vi "Destroy.vi"(8 "error in (no error)":errorcluster, 9 "ms Timeout (500)":u32=500, 11 "Queue in":refnum<queue>) -> (0 "error out":errorcluster, 1 "ms Elapsed":u32, 3 "Queue out":refnum<queue>)   [LabVIEW 2021, in "QueueTimer.lvlib"]
doc: "Destroys all queue timers associated with the <b>Queue</b> reference and stops the daemon threads. Specify the <b>ms Timeout</b> to wait for the daemon thread to close.\n\nNote: The Wait on Async is used which hardcodes the timeout values, supported timeout values are 0ms (No wait), 500ms, 2000ms and 5000ms."
uses:
  QueueTimer.lvlib
  <vilib>/Utility/error.llb/Error Cluster From Error Code.vi
  <vilib>/ErrorRing/Error Ring.xnode
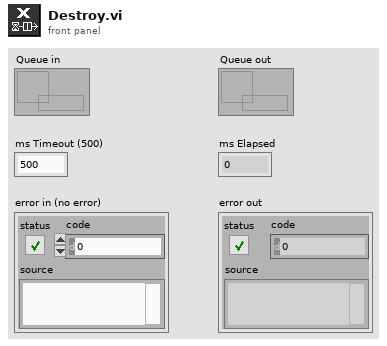
[diagram p1: front panel]
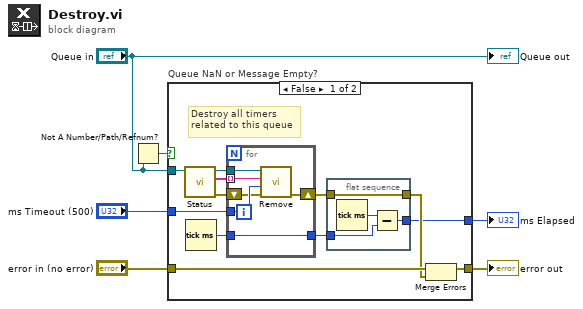
[diagram p0: block diagram]
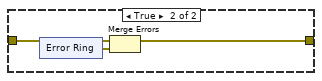
[diagram p2: hidden frame]
diagram:
  n1 = Not A Number/Path/Refnum?(number/path/refnum="Queue in") -> (NaN/Path/Refnum?=w3:bool)
  n2 = case "Queue NaN or Message Empty?" shown="False" w3 {
    tunnel: "Queue in" -> [w17 _]
    tunnel: "error in (no error)" -> [w10 w31]
    tunnel: [w13 w30] -> w5
    tunnel: "ms Timeout (500)" -> [w18 _]
    tunnel: [w7 _] -> w2
    frame False {
      # "Destroy all timers\nrelated to this queue"
      n3 = call "Status.vi"("Queue in"=w17) -> ("error out"=w15:errorcluster, "Timer Messages"=w14:string[], "Queue out"=w16:refnum<queue>)  [unwired: 5 in, 3 out]
      n4 = Tick Count (ms)() -> (millisecond timer value=w12:u32)
      n5 = for {
        tunnel: w18 -> [w27]
        tunnel: w16 -> [w26]
        tunnel: w14 -> [w24] mode=indexing
        shift-right: [w28] -> w8
        shift-left: w15 -> [w25]
        tunnel: [w23] -> w11
        tunnel: w12 -> [w23]
        n6 = call "Remove.vi"("error in (no error)"=w25, "ms Timeout (500)"=w27, "Timer Message"=w24, "Queue in"=w26) -> ("error out"=w28:errorcluster)  [unwired: 5 in, 2 out]
      }
      n7 = flat-sequence {
        tunnel: w11 -> [w21]
        tunnel: [w20] -> w9
        tunnel: w8 -> [w20]
        tunnel: [w19] -> w7
        frame #0 {
          n8 = Tick Count (ms)() -> (millisecond timer value=w22:u32)
          n9 = Subtract(x=w22, y=w21) -> (x-y=w19:u32)
        }
      }
      n10 = Merge Errors(w10, w9) -> (w13:errorcluster)
    }
    frame True {
      n11 = xnode "Error Ring"() -> ("error out"=w29:errorcluster)
      n12 = Merge Errors(w31, w29) -> (w30:errorcluster)
    }
  }
  "error out" <- w5
  "ms Elapsed" <- w2
  "Queue out" <- "Queue in"
